vi "Source_Voltage.vi"(4 "Source Delay (Sec)":dbl=0.1 format="%.3p", 6 "Current Limit Range":dbl=0.01 format="%.3p", 7 "Current Limit":dbl=0.01 format="%.3p", 8 "error in (no error)":errorcluster, 9 "Voltage Level Range":dbl=6.0 format="%.5p", 10 "Voltage Level":dbl=2.0 format="%.5p", 11 "Source_Voltage in":refnum<class "Source_Voltage.lvclass">) -> (0 "error out":errorcluster, 3 "Source_Voltage out":refnum<class "Source_Voltage.lvclass">)   [LabVIEW 2021, in "Source_Voltage.lvclass"]
uses:
  Source_Voltage.lvclass
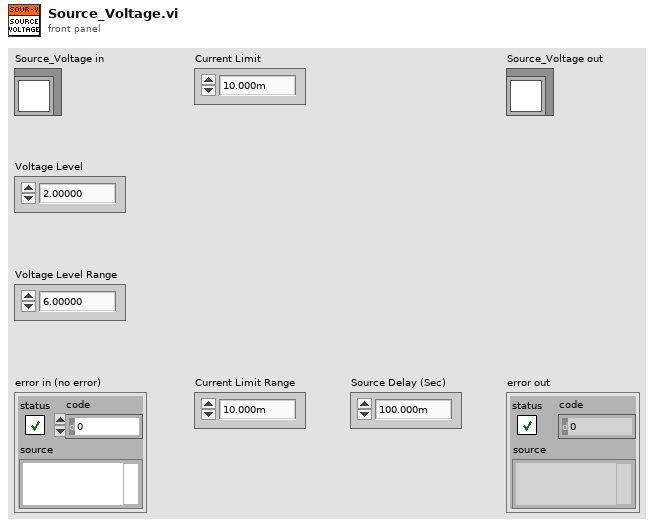
[diagram p1: front panel]
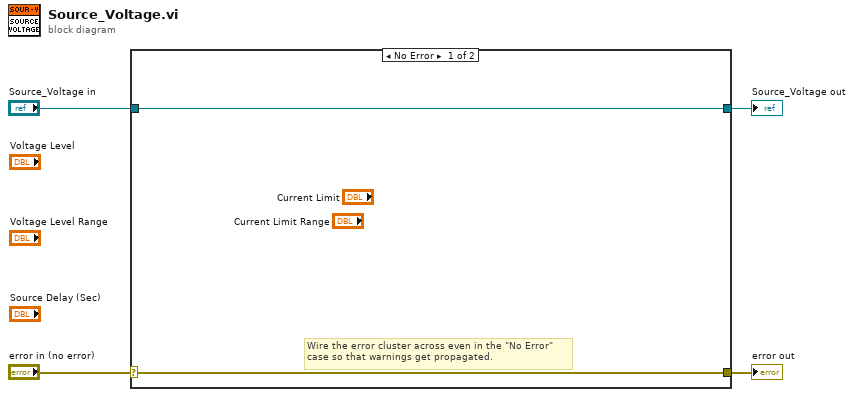
[diagram p0: block diagram]
diagram:
  n1 = case shown="No Error" "error in (no error)" {
    selector: "error in (no error)" -> [w5 w8]
    tunnel: [w5 w8] -> w3
    tunnel: [w6 w7] -> w1
    tunnel: "Source_Voltage in" -> [w6 w7]
    frame No Error {
      # "Wire the error cluster across even in the \"No Error\"\ncase so that warnings get propagated."
    }
    frame Error {
    }
  }
  "error out" <- w3
  "Source_Voltage out" <- w1
